vi "configure.vi"(0 "handle":u32, 5 "general":T2, 7 "runtime":T1, 9 "timing":cluster{"period":u32, "averaging":u8}, 11 "error in (no error)":errorcluster) -> (3 "function return":i32, 4 "handle out":u32, 6 "general out":T2, 8 "runtime out":T1, 10 "timing out":cluster{"period":u32, "averaging":u8}, 15 "error out":errorcluster)   [LabVIEW 2013]
doc: "EXPORT int buddy_configure(hid_device *handle, ctrl_general_t *general, ctrl_runtime_t *runtime, ctrl_timing_t *timing);"
uses:
  buddy/x64/Debug/buddy.dll
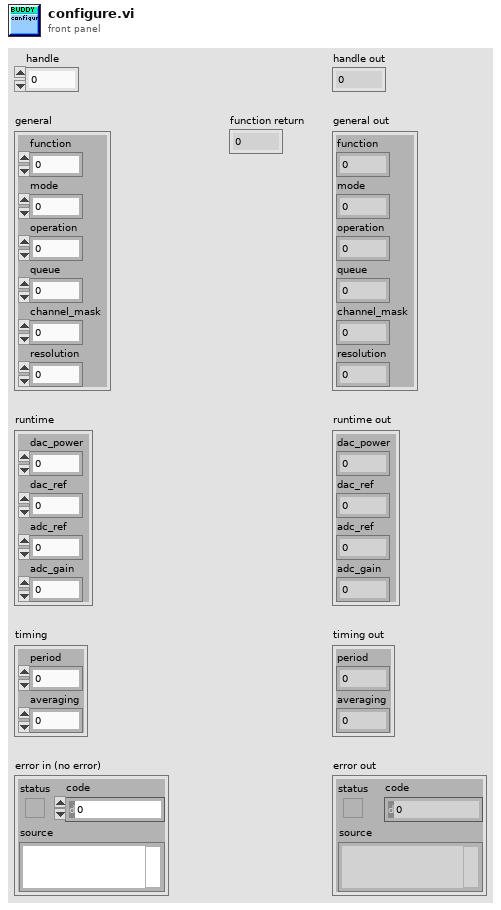
[diagram p1: front panel]
types:
  T1 = cluster{"dac_power":u8, "dac_ref":u8, "adc_ref":u8, "adc_gain":u8}
  T2 = cluster{"function":u8, "mode":u8, "operation":u8, "queue":u8, "channel_mask":u8, "resolution":u8}
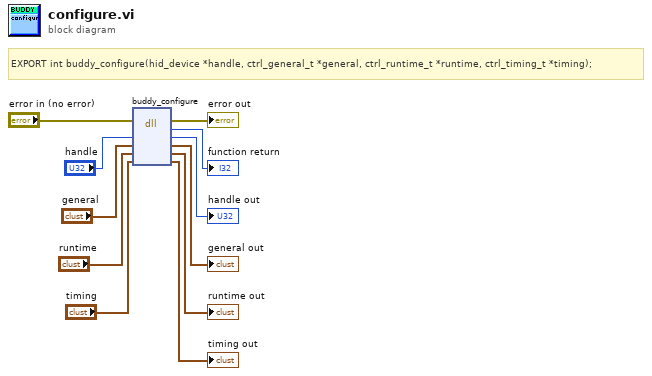
[diagram p0: block diagram]
diagram:
  # "EXPORT int buddy_configure(hid_device *handle, ctrl_general_t *general, ctrl_runtime_t *runtime, ctrl_timing_t *timing);"
  n1 = dll-call lib="C:/Users/shraken/shraken_code/usbhid_buddy/lib/libbuddy/bindings/labview/buddy/x64/Debug/buddy.dll" fn="buddy_configure"(error in="error in (no error)", "handle"="handle", "general"="general", "runtime"="runtime", "timing"="timing") -> (error out=→"error out":errorcluster, "return type"=→"function return":i32, "handle"=→"handle out":u32, "general"=→"general out":T2, "runtime"=→"runtime out":T1, "timing"=→"timing out":cluster{"period":u32, "averaging":u8})  [unwired: 2 in, 1 out]
